vi "DriveBase.vi"(9 "Elevator State":string="Hatch_Rocket_1") -> ()   [LabVIEW 2018]
uses:
  RobotStates.vi
  Inputs_DriverStation.vi
  SensorReadings.vi
  RefNums_DriverStation.vi
panel:
  in  "Forward Acceleration (p/s)":dbl=10.0
  in  "Time Above Speed (ms)":u32=100
  in  "Stabilization Height (in)":dbl=36.0
  in  "Switch to Low Gear (ft/s)":dbl=0.5
  in  "Switch to High Gear (ft/s)":dbl=6.0
  in  "Elevator Danger Height (in)":dbl=52.0
  in  "Backward Acceleration (p/s)":dbl=1.0
  in  "Climb-Drive Bias":dbl=-0.4
  in  "Turning Deadband":dbl=0.2
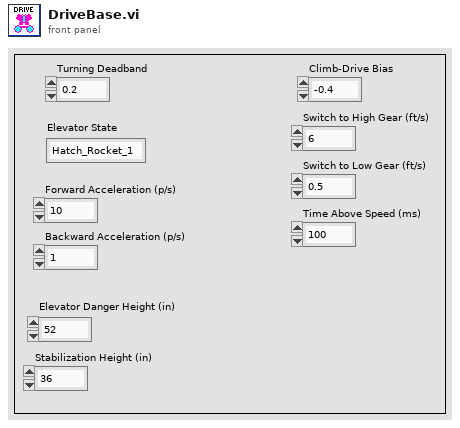
[diagram p1: front panel]
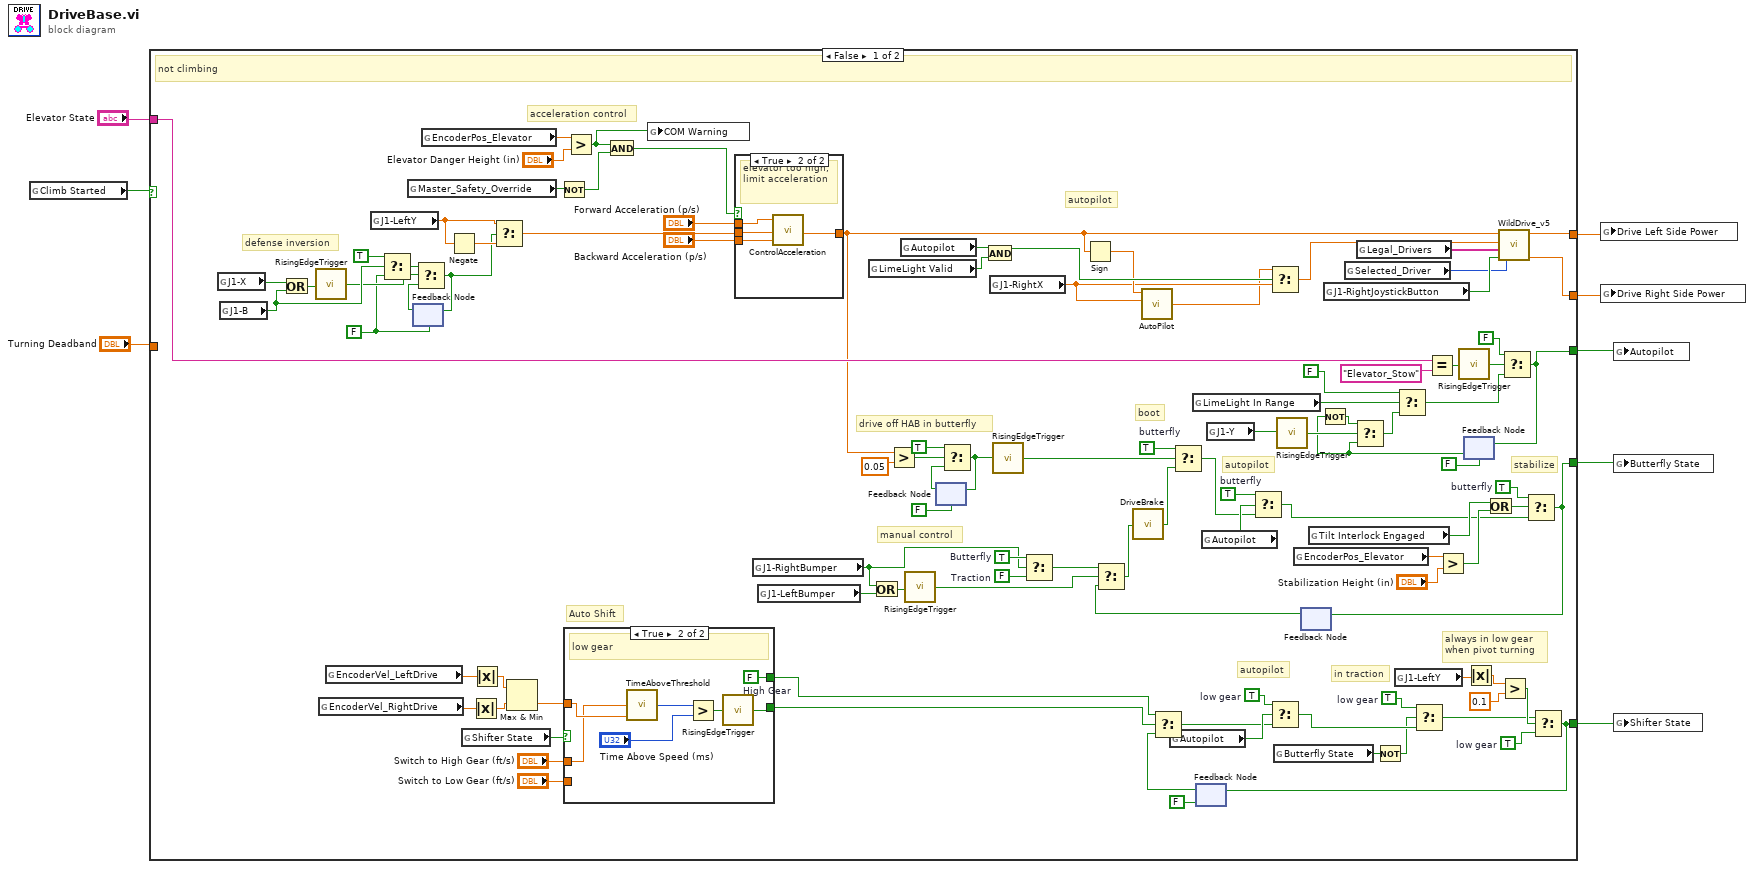
[diagram p0: block diagram]
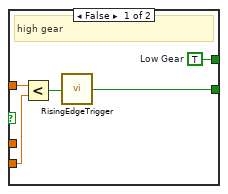
[diagram p2: hidden frame]
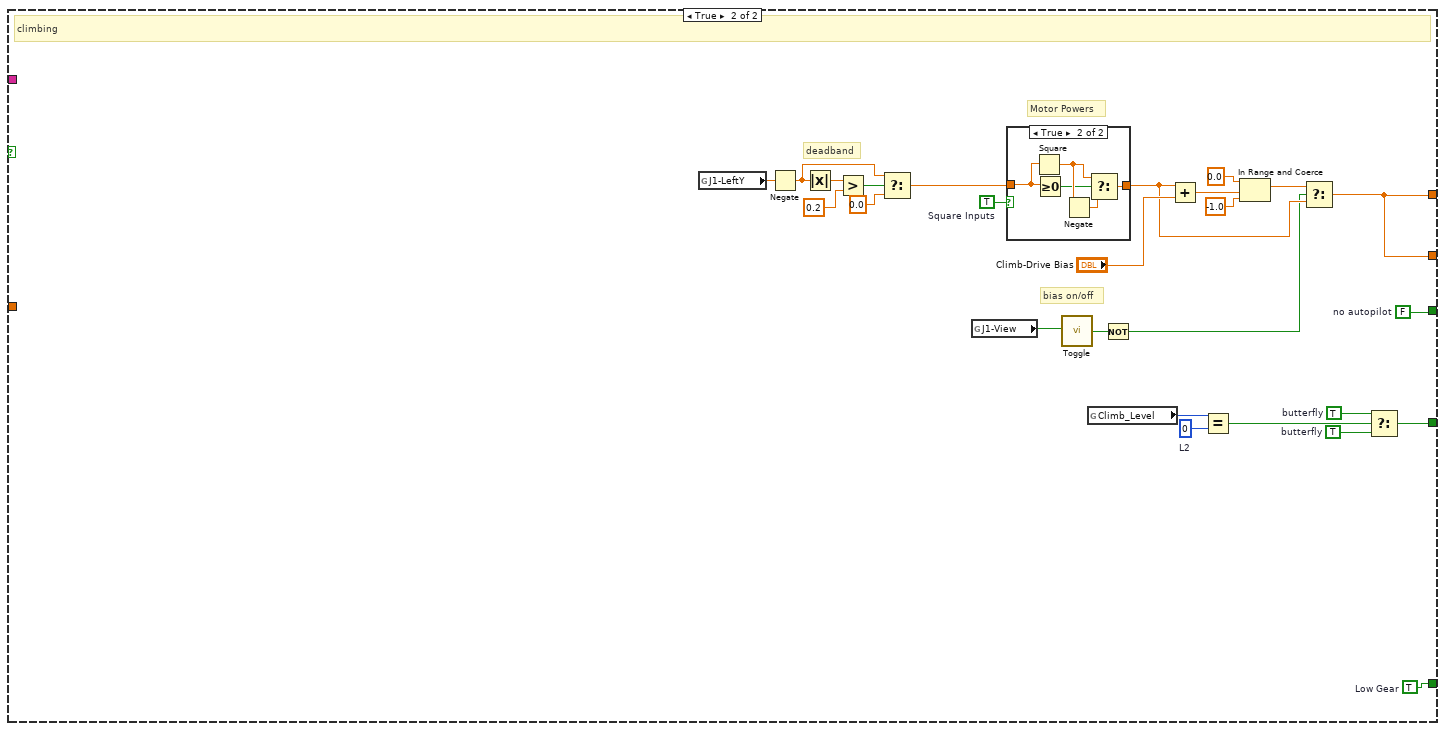
[diagram p4: hidden frame]
diagram:
  n1 = global read "RobotStates.vi" "Climb Started"() -> (w5:bool)
  n2 = case shown="False" w5 {
    tunnel: [w75 w135] -> w8
    tunnel: [w65 w154] -> w7
    tunnel: "Turning Deadband" -> [_ _]
    tunnel: [w17 w137] -> w1
    tunnel: [w16 w137] -> w2
    tunnel: [w44 w136] -> w4
    tunnel: "Elevator State" -> [w43 _]
    frame False {
      w21 = FALSE
      w33 = TRUE  # low gear
      w55 = TRUE  # butterfly
      w58 = TRUE  # low gear
      w64 = TRUE  # low gear
      w76 = FALSE  # Traction
      w77 = TRUE  # Butterfly
      w83 = TRUE  # butterfly
      w90 = TRUE  # butterfly
      # "defense inversion"
      # "in traction"
      # "acceleration control"
      # "always in low gear\nwhen pivot turning"
      # "autopilot"
      # "stabilize"
      # "autopilot"
      # "boot"
      # "manual control"
      # "autopilot"
      # "drive off HAB in butterfly"
      # "Auto Shift"
      # "not climbing"
      n3 = global read "Inputs_DriverStation.vi" "J1-X"() -> (w66:bool)
      n4 = global read "Inputs_DriverStation.vi" "J1-B"() -> (w26:bool)
      n5 = Or(x=w66, y=w26) -> (x .or. y?=w111:bool)
      n6 = call "RisingEdgeTrigger.vi"("Raw Signal"=w111) -> ("Trigger"=w23:bool)
      n7 = global read "SensorReadings.vi" "EncoderVel_RightDrive"() -> (w98:dbl)
      n8 = global read "SensorReadings.vi" "EncoderVel_LeftDrive"() -> (w99:dbl)
      n9 = global read "Inputs_DriverStation.vi" "J1-LeftY"() -> (w14:dbl)
      n10 = Select(t=TRUE, s=w26, f=w21) -> (s? t:f=w24:bool)
      n11 = global read "Inputs_DriverStation.vi" "Master_Safety_Override"() -> (w102:bool)
      n12 = feedback #1(w21) -> (w22:bool)
      n13 = Select(t=w24, s=w23, f=w22) -> (s? t:f=w12:bool)
      n14 = feedback-in #1(w12) -> ()
      n15 = global read "SensorReadings.vi" "EncoderPos_Elevator"() -> (w105:dbl)
      n16 = Negate(x=w14) -> (-x=w15:dbl)
      n17 = global read "RobotStates.vi" "Shifter State"() -> (w97:bool)
      n18 = Absolute Value(x=w98) -> (abs(x)=w92:dbl)
      n19 = Absolute Value(x=w99) -> (abs(x)=w93:dbl)
      n20 = Select(t=w14, s=w12, f=w15) -> (s? t:f=w20:dbl)
      n21 = Max & Min(x=w93, y=w92) -> (min(x,y)=w71:dbl)  [unwired: 1 out]
      n22 = Not(x=w102) -> (.not. x?=w101:bool)
      n23 = case shown="True" w97 {
        tunnel: w71 -> [w116 w118]
        tunnel: "Switch to High Gear (ft/s)" -> [_ w117]
        tunnel: "Switch to Low Gear (ft/s)" -> [w115 _]
        tunnel: [w112 w122] -> w91
        tunnel: [w114 w123] -> w94
        frame False {
          w114 = TRUE  # Low Gear
          # "high gear"
          n24 = Less?(x=w116, y=w115) -> (x < y?=w113:bool)
          n25 = call "RisingEdgeTrigger.vi"("Raw Signal"=w113) -> ("Trigger"=w112:bool)
        }
        frame True {
          w123 = FALSE  # High Gear
          # "low gear"
          n26 = call "TimeAboveThreshold.vi"("Current Value"=w118, "Threshold"=w117) -> ("Time Above"=w121:u32)  [unwired: 3 in]
          n27 = Greater?(x=w121, y="Time Above Speed (ms)") -> (0:w119:bool)
          n28 = call "RisingEdgeTrigger.vi"("Raw Signal"=w119) -> ("Trigger"=w122:bool)
        }
      }
      n29 = Greater?(x=w105, y="Elevator Danger Height (in)") -> (0:w100:bool)
      n30 = And(x=w100, y=w101) -> (x .and. y?=w103:bool)
      n31 = global write "RobotStates.vi" "COM Warning"(w100) -> ()
      n32 = case shown="True" w103 {
        tunnel: w20 -> [w124 w128]
        tunnel: [w124 w127] -> w19
        tunnel: "Backward Acceleration (p/s)" -> [_ w126]
        tunnel: "Forward Acceleration (p/s)" -> [_ w125]
        frame False {
          # "elevator down"
        }
        frame True {
          # "elevator too high, limit acceleration"
          n33 = call "ControlAcceleration.vi"("Backward Acceleration (p/s)"=w126, "Raw"=w128, "Forward Acceleration (p/s)"=w125) -> ("Controlled"=w127:dbl)
        }
      }
      n34 = global read "Inputs_DriverStation.vi" "J1-RightBumper"() -> (w73:bool)
      n35 = global read "Inputs_DriverStation.vi" "J1-LeftBumper"() -> (w74:bool)
      n36 = global read "SensorReadings.vi" "LimeLight Valid"() -> (w107:bool)
      n37 = Or(x=w73, y=w74) -> (x .or. y?=w81:bool)
      n38 = Greater?(x=w19, y=0.05) -> (0:w85:bool)
      n39 = global read "RobotStates.vi" "Autopilot"() -> (w109:bool)
      n40 = call "RisingEdgeTrigger.vi"("Raw Signal"=w81) -> ("Trigger"=w78:bool)
      n41 = feedback #2(FALSE) -> (w88:bool)
      n42 = Select(t=TRUE, s=w85, f=w88) -> (s? t:f=w87:bool)
      n43 = feedback-in #2(w87) -> ()
      n44 = And(x=w109, y=w107) -> (x .and. y?=w108:bool)
      n45 = global read "Inputs_DriverStation.vi" "J1-RightX"() -> (w28:dbl)
      n46 = call "RisingEdgeTrigger.vi"("Raw Signal"=w87) -> ("Trigger"=w72:bool)
      n47 = Select(t=w77, s=w73, f=w76) -> (s? t:f=w79:bool)
      n48 = Sign(1:w19) -> (0:w52:dbl)
      n49 = call "AutoPilot.vi"("Human Contribution"=w28, "Drive Direction"=w52) -> ("End Contribution"=w13:dbl)  [unwired: 2 in]
      n50 = global read "RobotStates.vi" "Autopilot"() -> (w59:bool)
      n51 = global read "SensorReadings.vi" "LimeLight In Range"() -> (w36:bool)
      n52 = feedback #3(FALSE ("Low Gear")) -> (w27:bool)
      n53 = Select(t=w94, s=w91, f=w27) -> (s? t:f=w57:bool)
      n54 = global read "RobotStates.vi" "Autopilot"() -> (w56:bool)
      n55 = global read "Inputs_DriverStation.vi" "J1-Y"() -> (w45:bool)
      n56 = Select(t=w13, s=w108, f=w28) -> (s? t:f=w18:dbl)
      n57 = Select(t=w58, s=w59, f=w57) -> (s? t:f=w32:bool)
      n58 = global read "RobotStates.vi" "Butterfly State"() -> (w30:bool)
      n59 = call "RisingEdgeTrigger.vi"("Raw Signal"=w45) -> ("Trigger"=w48:bool)
      n60 = global read "SensorReadings.vi" "EncoderPos_Elevator"() -> (w70:dbl)
      n61 = feedback #4() -> (w80:bool)  [unwired: 1 in]
      n62 = Select(t=w79, s=w78, f=w80) -> (s? t:f=w38:bool)
      n63 = call "DriveBrake.vi"("Butterfly State In"=w38) -> ("Butterfly State Out"=w39:bool)
      n64 = Select(t=w90, s=w72, f=w39) -> (s? t:f=w54:bool)
      n65 = Select(t=w55, s=w56, f=w54) -> (s? t:f=w53:bool)
      n66 = global read "RobotStates.vi" "Tilt Interlock Engaged"() -> (w67:bool)
      n67 = global read "Inputs_DriverStation.vi" "J1-RightJoystickButton"() -> (w11:bool)
      n68 = global read "Inputs_DriverStation.vi" "Selected_Driver"() -> (w9:i32)
      n69 = global read "RefNums_DriverStation.vi" "Legal_Drivers"() -> (w10:string[])
      n70 = Not(x=w30) -> (.not. x?=w29:bool)
      n71 = global read "Inputs_DriverStation.vi" "J1-LeftY"() -> (w63:dbl)
      n72 = Select(t=w33, s=w29, f=w32) -> (s? t:f=w31:bool)
      n73 = Equal?(x=w43, y="Elevator_Stow") -> (x = y?=w41:bool)
      n74 = Greater?(x=w70, y="Stabilization Height (in)") -> (0:w68:bool)
      n75 = call "RisingEdgeTrigger.vi"("Raw Signal"=w41) -> ("Trigger"=w40:bool)
      n76 = feedback #5(FALSE) -> (w46:bool)
      n77 = Not(x=w46) -> (.not. x?=w47:bool)
      n78 = Select(t=w47, s=w48, f=w46) -> (s? t:f=w35:bool)
      n79 = Select(t=FALSE, s=w36, f=w35) -> (s? t:f=w34:bool)
      n80 = Absolute Value(x=w63) -> (abs(x)=w62:dbl)
      n81 = Or(x=w67, y=w68) -> (x .or. y?=w82:bool)
      n82 = call "WildDrive_v5.vi"("Selected_Driver"=w9, "Super Turn"=w11, "Legal_Drivers"=w10, "Turn Joystick"=w18, "Speed Joystick"=w19) -> ("Right Side Power"=w16:dbl, "Left Side Power"=w17:dbl)  [unwired: 5 in]
      n83 = Greater?(x=w62, y=0.1) -> (0:w61:bool)
      n84 = Select(t=FALSE, s=w40, f=w34) -> (s? t:f=w44:bool)
      n85 = feedback-in #5(w44) -> ()
      n86 = Select(t=w83, s=w82, f=w53) -> (s? t:f=w75:bool)
      n87 = feedback-in #4(w75) -> ()
      n88 = Select(t=w31, s=w61, f=w64) -> (s? t:f=w65:bool)
      n89 = feedback-in #3(w65) -> ()
    }
    frame True {
      w131 = u8 0  # L2
      w133 = TRUE  # butterfly
      w136 = FALSE  # no autopilot
      w148 = TRUE  # Square Inputs
      w154 = TRUE  # Low Gear
      w134 = TRUE  # butterfly
      # "deadband"
      # "bias on/off"
      # "Motor Powers"
      # "climbing"
      n90 = global read "Inputs_DriverStation.vi" "J1-LeftY"() -> (w151:dbl)
      n91 = Negate(x=w151) -> (-x=w152:dbl)
      n92 = Absolute Value(x=w152) -> (abs(x)=w149:dbl)
      n93 = Greater?(x=w149, y=0.2) -> (0:w150:bool)
      n94 = Select(t=w152, s=w150, f=0.0) -> (s? t:f=w153:dbl)
      n95 = global read "Inputs_DriverStation.vi" "J1-View"() -> (w142:bool)
      n96 = case shown="True" w148 {
        tunnel: [w155 w160] -> w139
        tunnel: w153 -> [w155 w159]
        frame False {
        }
        frame True {
          n97 = Square(x=w159) -> (x^2=w157:dbl)
          n98 = Greater Or Equal To 0?(x=w159) -> (x >= 0?=w156:bool)
          n99 = Negate(x=w157) -> (-x=w158:dbl)
          n100 = Select(t=w157, s=w156, f=w158) -> (s? t:f=w160:dbl)
        }
      }
      n101 = call "Toggle.vi"("Trigger"=w142) -> ("New Mode"=w141:bool)
      n102 = global read "Inputs_DriverStation.vi" "Climb_Level"() -> (w132:u8)
      n103 = Not(x=w141) -> (.not. x?=w138:bool)
      n104 = Add(x=w139, y="Climb-Drive Bias") -> (x+y=w146:dbl)
      n105 = Equal?(x=w132, y=w131) -> (x = y?=w130:bool)
      n106 = In Range and Coerce(upper limit=0.0, x=w146, lower limit=-1.0) -> (coerced(x)=w140:dbl)  [unwired: 1 out]
      n107 = Select(t=w140, s=w138, f=w139) -> (s? t:f=w137:dbl)
      n108 = Select(t=w133, s=w130, f=w134) -> (s? t:f=w135:bool)
    }
  }
  n109 = global write "RobotStates.vi" "Drive Left Side Power"(w1) -> ()
  n110 = global write "RobotStates.vi" "Drive Right Side Power"(w2) -> ()
  n111 = global write "RobotStates.vi" "Autopilot"(w4) -> ()
  n112 = global write "RobotStates.vi" "Butterfly State"(w8) -> ()
  n113 = global write "RobotStates.vi" "Shifter State"(w7) -> ()
